vi "BuildPython.vi"(9 "Subscriber":T1={"Node Name"="Node", "Topic Name"="/cmd_lightring", "Message Type"="irobot_create_msgs/msg/LightringLeds", "Message"="{\"override_system\":true,\"leds\":[{\"red\":255,\"green\":0,\"blue\":0},{\"red\":4,\"green\":255,\"blue\":0},{\"red\":6,\"green\":0,\"blue\":255},{\"red\":239,\"green\":142,\"blue\":0},{\"red\":226,\"green\":0,\"blue\":255},{\"red\":0,\"green\":250,\"blue\":255}]}", "Pub_Time"="-1"}, 11 "Publisher":T1={"Node Name"="Node", "Topic Name"="/cmd_lightring", "Message Type"="irobot_create_msgs/msg/LightringLeds", "Message"="{\"override_system\":true,\"leds\":[{\"red\":255,\"green\":0,\"blue\":0},{\"red\":4,\"green\":255,\"blue\":0},{\"red\":6,\"green\":0,\"blue\":255},{\"red\":239,\"green\":142,\"blue\":0},{\"red\":226,\"green\":0,\"blue\":255},{\"red\":0,\"green\":250,\"blue\":255}]}", "Pub_Time"="5"}) -> (0 "result both":string, 1 "result Sub":string, 3 "result Pub":string="import rclpy\nfrom rclpy.node import Node\n\nfrom irobot_create_msgs.msg import LedColor\nimport irobot_create_msgs\n\nclass myPublisher(Node):\n    ''' Publish a custom color to each LED on the Create3 '''\n\n    def __init__(self, namespace: str = \"\"):\n        super().__init__('Node')\n        self.publisher = self.create_publisher(irobot_create_msgs.msg.LightringLeds, namespace + '/cmd_lightring', 10)\n\n        timer_period = 5 # seconds\n        self.timer = self.create_timer(timer_period, self.timer_callback)\n        self.payload = irobot_create_msgs.msg.LightringLeds()\n\n    def timer_callback(self):\n        '''This function will be called every 5 seconds '''\n        current_time = self.get_clock().now()\n\n        c0 = LedColor(red=255, green=0, blue=0)\n        c1 = LedColor(red=4, green=255, blue=0)\n        c2 = LedColor(red=6, green=0, blue=255)\n        c3 = LedColor(red=239, green=142, blue=0)\n        c4 = LedColor(red=226, green=0, blue=255)\n        c5 = LedColor(red=0, green=250, blue=255)\n        self.payload.override_system = True\n        self.payload.leds = [c0,c1,c2,c3,c4,c5]\n\n        self.payload.header.stamp = current_time.to_msg()\n        self.publisher.publish(self.payload)\n\ndef main():\n    rclpy.init()\n    publisher = myPublisher()\n\n    try:\n        rclpy.spin(publisher)\n    except KeyboardInterrupt:\n        print('\\nCaught Keyboard Interrupt')\n    finally:\n        print(\"Done\")\n        publisher.reset()\n        publisher.destroy_node()\n        rclpy.shutdown()\n\nmain()")   [LabVIEW 2021]
uses:
  ROSCtrl.ctl
panel:
  in  "Tab Control":enum32{"Pub", "Sub", "Both"}(tab)
  # "-1 means \nsubscribe"
  # "-1 means \nsubscribe"
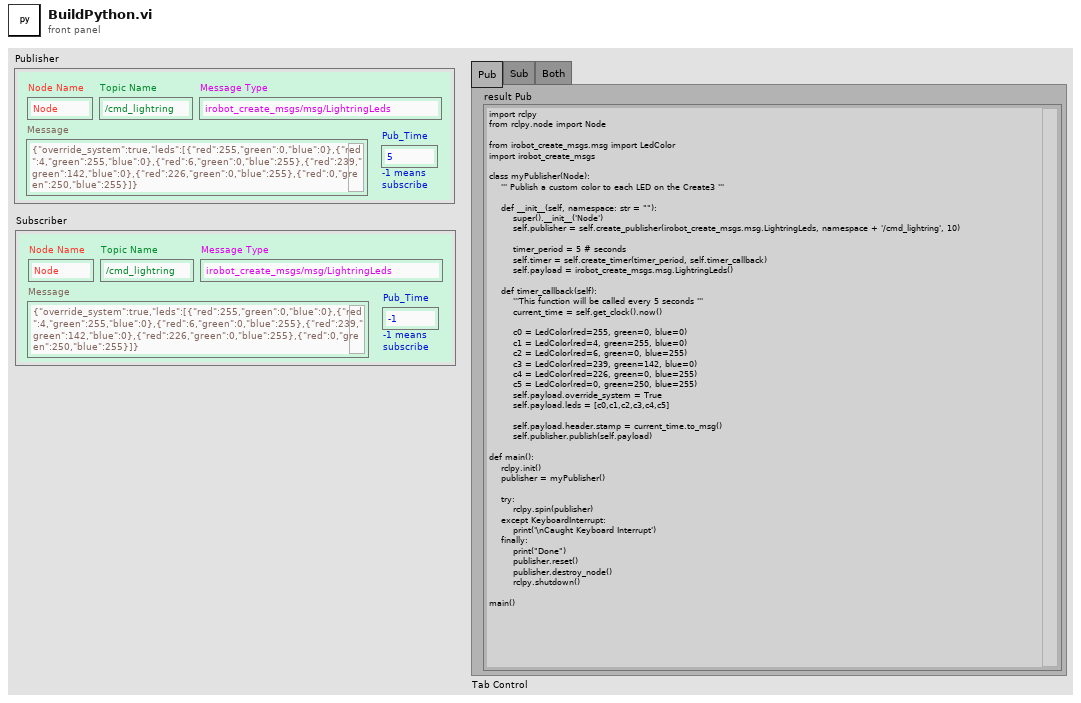
[diagram p1: front panel]
types:
  T1 = typedef "ROSCtrl.ctl" = cluster{"Node Name":string, "Topic Name":string, "Message Type":string, "Message":string, "Pub_Time":string}
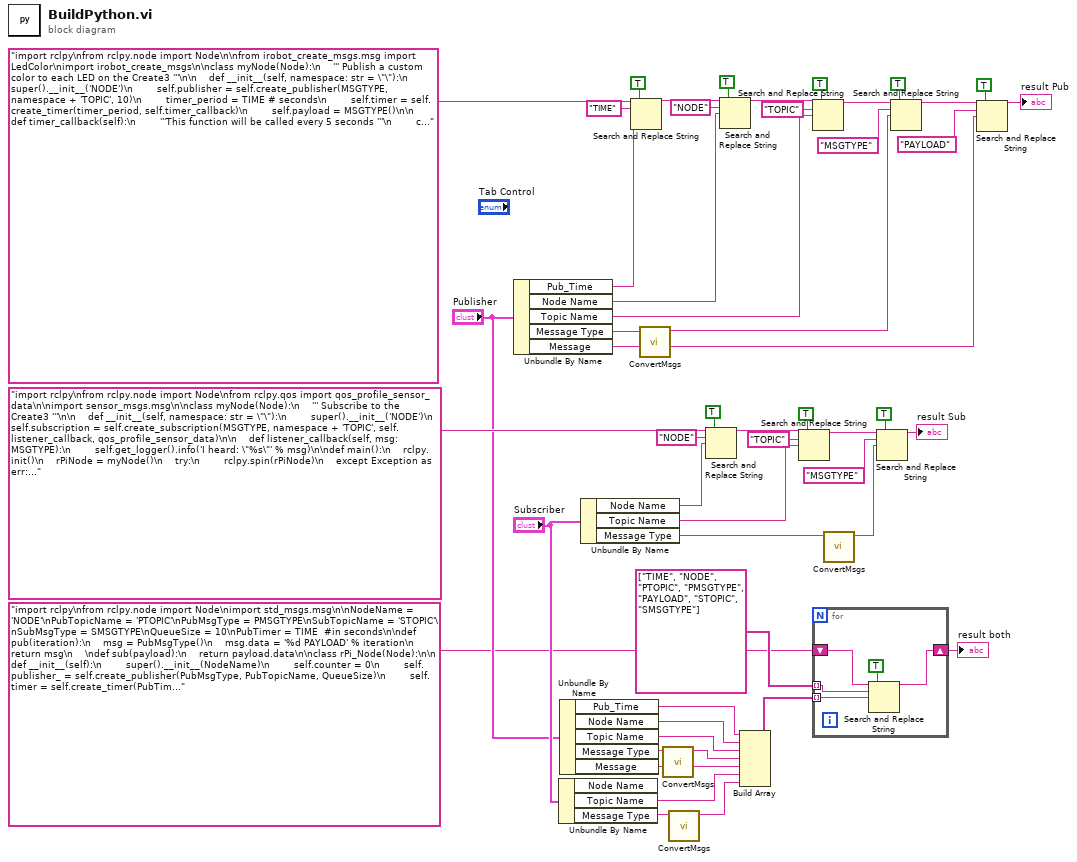
[diagram p0: block diagram]
diagram:
  n1 = Unbundle By Name("Publisher") -> ("Pub_Time"=w34:string, "Node Name"=w35:string, "Topic Name"=w33:string, "Message Type"=w4:string, "Message"=w32:string)
  n2 = Unbundle By Name("Subscriber") -> ("Topic Name"=w11:string, "Message Type"=w10:string)  [unwired: 1 out]
  n3 = Unbundle By Name("Publisher") -> ("Pub_Time"=w16:string, "Node Name"=w15:string, "Topic Name"=w14:string, "Message Type"=w19:string, "Message"=w12:string)
  n4 = Unbundle By Name("Subscriber") -> ("Node Name"=w30:string, "Topic Name"=w31:string, "Message Type"=w2:string)
  n5 = Search and Replace String(replace all?=TRUE ("replace all? (F)"), input string="import rclpy\nfrom rclpy.node import Node\n\nfrom irobot_create_msgs.msg import LedColor\nimport irobot_create_msgs\n\nclass myNode(Node):\n    ''' Publish a custom color to each LED on the Create3 '''\n\n    def __init__(self, namespace: str = \"\"):\n        super().__init__('NODE')\n        self.publisher = self.create_publisher(MSGTYPE, namespace + 'TOPIC', 10)\n        timer_period = TIME # seconds\n        self.timer = self.create_timer(timer_period, self.timer_callback)\n        self.payload = MSGTYPE()\n\n    def timer_callback(self):\n        '''This function will be called every 5 seconds '''\n        current_time = self.get_clock().now()\n\nPAYLOAD\n        self.payload.header.stamp = current_time.to_msg()\n        self.publisher.publish(self.payload)\n\ndef main():\n    rclpy.init()\n    rPiNode = myNode()\n\n    try:\n        rclpy.spin(rPiNode)\n    except Exception as err:\n        print(err)\n    finally:\n        #rPiNode.reset()\n        rPiNode.destroy_node()\n        rclpy.shutdown()\n        print(\"Done\")\nmain()" ("Python"), search string="TIME", replace string=w34) -> (result string=w36:string)  [unwired: 4 in, 3 out]
  n6 = call "ConvertMsgs.vi"("Message Type"=w4) -> ("result string"=w3:string)  [unwired: 10 in]
  n7 = call "ConvertMsgs.vi"("Message Type"=w19) -> ("result string"=w13:string)  [unwired: 10 in]
  n8 = call "ConvertMsgs.vi"("Message Type"=w10) -> ("result string"=w9:string)  [unwired: 10 in]
  n9 = Search and Replace String(replace all?=TRUE ("replace all? (F)"), input string="import rclpy\nfrom rclpy.node import Node\nfrom rclpy.qos import qos_profile_sensor_data\n\nimport sensor_msgs.msg\n\nclass myNode(Node):\n    ''' Subscribe to the Create3 '''\n\n    def __init__(self, namespace: str = \"\"):\n        super().__init__('NODE')\n        self.subscription = self.create_subscription(MSGTYPE, namespace + 'TOPIC', self.listener_callback, qos_profile_sensor_data)\n\n    def listener_callback(self, msg: MSGTYPE):\n        self.get_logger().info('I heard: \"%s\"' % msg)\n\ndef main():\n    rclpy.init()\n    rPiNode = myNode()\n    try:\n        rclpy.spin(rPiNode)\n    except Exception as err:\n        print(err)\n    finally:\n        #rPiNode.reset()\n        rPiNode.destroy_node()\n        rclpy.shutdown()\n        print(\"Done\")\nmain()" ("Python"), search string="NODE", replace string=w30) -> (result string=w26:string)  [unwired: 4 in, 3 out]
  n10 = Search and Replace String(replace all?=TRUE ("replace all? (F)"), input string=w36, search string="NODE", replace string=w35) -> (result string=w47:string)  [unwired: 4 in, 3 out]
  n11 = Build Array(w16, w15, w14, w13, w12, w11, w9) -> (w7:string[])
  n12 = Search and Replace String(replace all?=TRUE ("replace all? (F)"), input string=w26, search string="TOPIC", replace string=w31) -> (result string=w29:string)  [unwired: 4 in, 3 out]
  n13 = Search and Replace String(replace all?=TRUE ("replace all? (F)"), input string=w47, search string="TOPIC", replace string=w33) -> (result string=w44:string)  [unwired: 4 in, 3 out]
  n14 = for {
    shift-right: [w54] -> w5
    shift-left: "import rclpy\nfrom rclpy.node import Node\nimport std_msgs.msg\n\nNodeName = 'NODE'\nPubTopicName = 'PTOPIC'\nPubMsgType = PMSGTYPE\nSubTopicName = 'STOPIC'\nSubMsgType = SMSGTYPE\nQueueSize = 10\nPubTimer = TIME  #in seconds\n\ndef pub(iteration):\n    msg = PubMsgType()\n    msg.data = '%d PAYLOAD' % iteration\n    return msg\n    \ndef sub(payload):\n    return payload.data\n\nclass rPi_Node(Node):\n\n    def __init__(self):\n        super().__init__(NodeName)\n        self.counter = 0\n        self.publisher_ = self.create_publisher(PubMsgType, PubTopicName, QueueSize)\n        self.timer = self.create_timer(PubTimer, self.pub_cb)\n        self.subscription = self.create_subscription(SubMsgType, SubTopicName, self.sub_cb, QueueSize)\n        self.subscription  # prevent unused variable warning\n        \n    def sub_cb(self, msg):\n        payload = sub(msg)\n        self.get_logger().info('Received: \"%s\"' % payload)\n\n    def pub_cb(self):\n        payload = pub(self.counter)\n        self.publisher_.publish(payload)\n        self.get_logger().info('Published: \"%s\"' % payload.data) #write to console\n        self.counter += 1\n\ndef main():\n    try:\n        rclpy.init()\n        myNode  = rPi_Node()\n        rclpy.spin(myNode)\n    except Exception as err:\n        print(err)\n    finally:\n        myNode.destroy_node()\n        rclpy.shutdown()\nmain()\n" ("Python") -> [w55]
    tunnel: string[] ["TIME", "NODE", "PTOPIC", "PMSGTYPE", "PAYLOAD", "STOPIC", "SMSGTYPE"] -> [w53] mode=indexing
    tunnel: w7 -> [w52] mode=indexing
    n15 = Search and Replace String(replace all?=TRUE ("replace all? (F)"), input string=w55, search string=w53, replace string=w52) -> (result string=w54:string)  [unwired: 4 in, 3 out]
  }
  "result both" <- w5
  n16 = call "ConvertMsgs.vi"("Message Type"=w2) -> ("result string"=w1:string)  [unwired: 10 in]
  n17 = Search and Replace String(replace all?=TRUE ("replace all? (F)"), input string=w29, search string="MSGTYPE", replace string=w1) -> (result string=→"result Sub":string)  [unwired: 4 in, 3 out]
  n18 = Search and Replace String(replace all?=TRUE ("replace all? (F)"), input string=w44, search string="MSGTYPE", replace string=w3) -> (result string=w41:string)  [unwired: 4 in, 3 out]
  n19 = Search and Replace String(replace all?=TRUE ("replace all? (F)"), input string=w41, search string="PAYLOAD", replace string=w32) -> (result string=→"result Pub":string)  [unwired: 4 in, 3 out]
